vi "Construct Close VIPM Step.vi"(5 "Close VIPM Step in":refnum<class "Close VIPM Step.lvclass">, 8 "error in (no error)":errorcluster) -> (0 "error out":errorcluster, 3 "Close VIPM Step":refnum<class "Close VIPM Step.lvclass">)   [LabVIEW 2019, in "VIPM.lvlib" / "Close VIPM Step.lvclass"]
uses:
  Close VIPM Step.lvclass
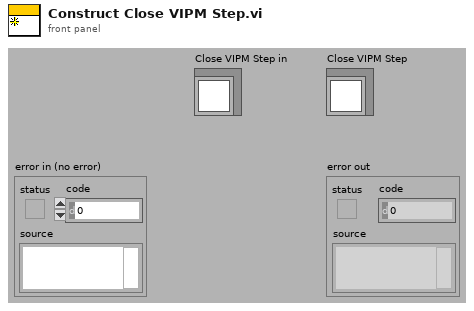
[diagram p1: front panel]
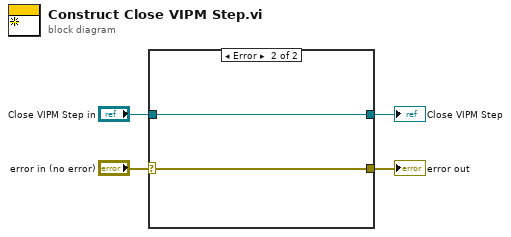
[diagram p0: block diagram]
diagram:
  n1 = case shown="Error" "error in (no error)" {
    selector: "error in (no error)" -> [w6 w8]
    tunnel: [w6 w8] -> w3
    tunnel: [w5 w7] -> w1
    tunnel: "Close VIPM Step in" -> [w5 w7]
    frame No Error {
    }
    frame Error {
    }
  }
  "error out" <- w3
  "Close VIPM Step" <- w1
